vi "sub UI set b.vi"(8 "error in (no error)":errorcluster, 10 "<b> data":T1, 11 "IDE simple in":refnum<class "LF2R IDE.lvclass">) -> (0 "error out":errorcluster, 3 "IDE simple out":refnum<class "LF2R IDE.lvclass">)   [LabVIEW 2018, in "LF2R IDE.lvlib" / "LF2R IDE.lvclass"]
uses:
  LF2R IDE.lvclass
  Frame Analizer/frame b data.ctl
  LF2R IDE.lvclass/LF2R IDE.ctl
  Frame Analizer/Frame Analizer.lvclass
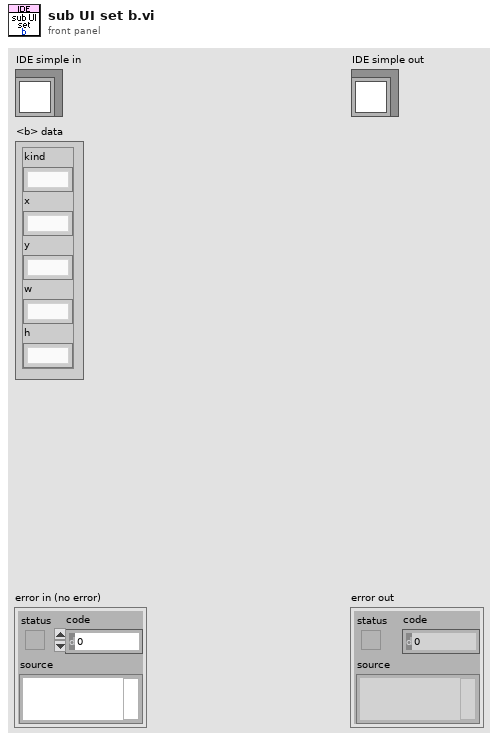
[diagram p1: front panel]
types:
  T1 = typedef "Frame Analizer.lvclass/frame b data.ctl" = cluster{"kind":string, "x":string, "y":string, "w":string, "h":string}
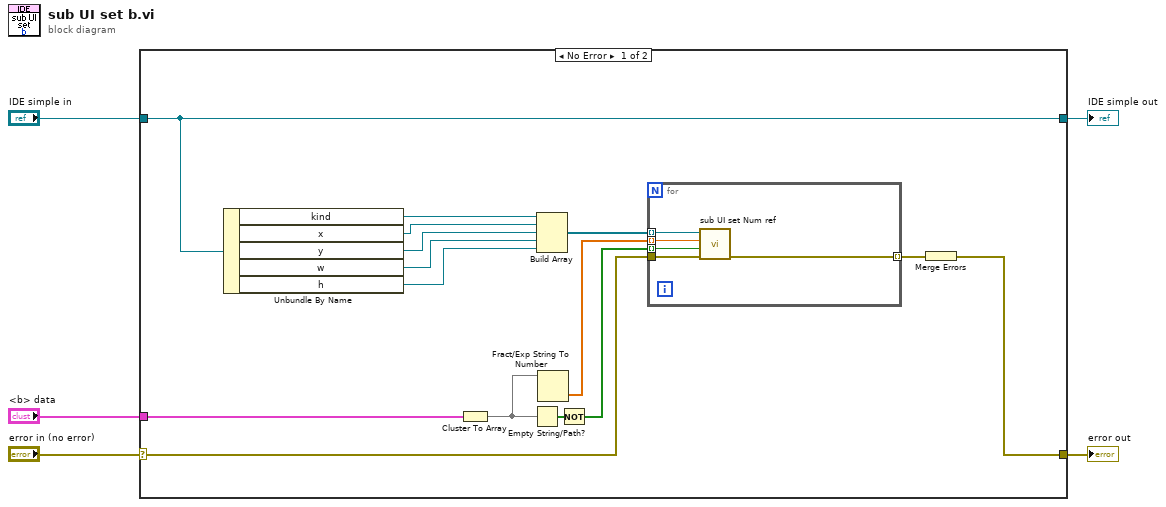
[diagram p0: block diagram]
diagram:
  n1 = case shown="No Error" "error in (no error)" {
    selector: "error in (no error)" -> [w19 w27]
    tunnel: [w14 w27] -> w4
    tunnel: [w16 w26] -> w2
    tunnel: "IDE simple in" -> [w16 w26]
    tunnel: "<b> data" -> [w13 _]
    frame No Error {
      n2 = Unbundle By Name(w16) -> ("kind"=w10:refnum<vi>, "x"=w9:refnum<vi>, "y"=w8:refnum<vi>, "w"=w7:refnum<vi>, "h"=w6:refnum<vi>)
      n3 = Cluster To Array(cluster=w13) -> (array=w12:string[])
      n4 = Empty String/Path?(string/path=w12) -> (empty?=w20:bool[])
      n5 = Build Array(w10, w9, w8, w7, w6) -> (w11:refnum<vi>[])
      n6 = Fract/Exp String To Number(string=w12) -> (number=w17:dbl[])  [unwired: 3 in, 1 out]
      n7 = Not(x=w20) -> (.not. x?=w18:bool[])
      n8 = for {
        tunnel: w19 -> [w25]
        tunnel: w11 -> [w21] mode=indexing
        tunnel: w18 -> [w22] mode=indexing
        tunnel: w17 -> [w24] mode=indexing
        tunnel: [w23] -> w15 mode=indexing
        n9 = call "sub UI set Num ref.vi"("error in"=w25, "valid"=w22, "Value"=w24, "num ref"=w21) -> ("error out"=w23:errorcluster)  [unwired: 7 in]
      }
      n10 = Merge Errors(w15) -> (w14:errorcluster)
    }
    frame Error {
    }
  }
  "error out" <- w4
  "IDE simple out" <- w2
